vi "save_txt.vi"(8 "error in (no error)":errorcluster, 10 "Data":dbl[](array[numeric]), 11 "Path":path) -> (0 "error out":errorcluster)   [LabVIEW 2024]
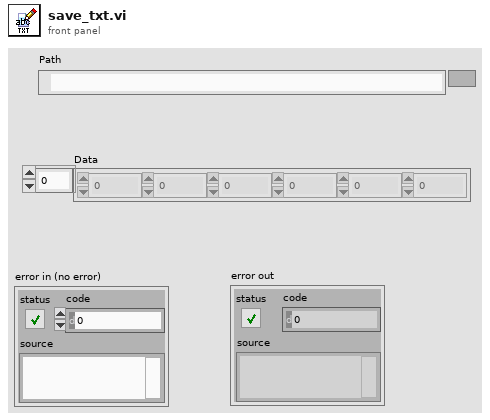
[diagram p1: front panel]
types:
  T1 = enum16{"open", "replace", "create", "open or create", "replace or create", "replace or create with confirmation"}
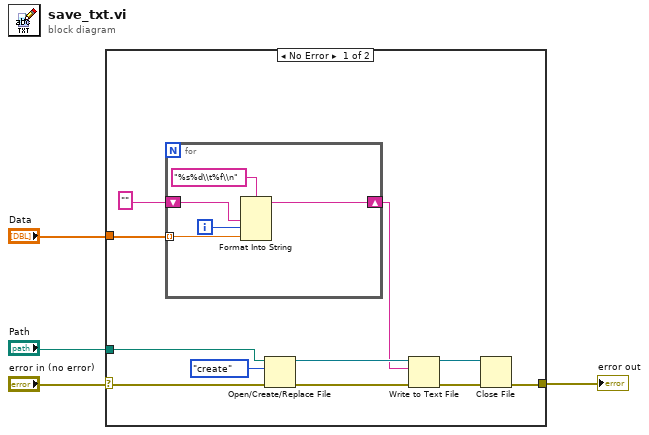
[diagram p0: block diagram]
diagram:
  n1 = case shown="No Error" "error in (no error)" {
    selector: "error in (no error)" -> [w14 w21]
    tunnel: [w11 w21] -> w3
    tunnel: "Data" -> [w15 _]
    tunnel: "Path" -> [w10 _]
    frame No Error {
      n2 = for {
        tunnel: w15 -> [w20] mode=indexing
        shift-right: [w18] -> w7
        shift-left: "" -> [w16]
        i -> [w17]
        n3 = Format Into String(format string="%s%d\\t%f\\n", w16, w17, w20) -> (resulting string=w18:string)  [unwired: 2 in, 1 out]
      }
      n4 = Open/Create/Replace File(file path (use dialog)=w10, error in=w14, operation (0:open)=T1."create") -> (refnum out=w9:refnum<file>, error out=w13:errorcluster)  [unwired: 3 in, 1 out]
      n5 = Write to Text File(file (use dialog)=w9, text=w7, error in=w13) -> (refnum out=w8:refnum<file>, error out=w12:errorcluster)  [unwired: 1 in, 1 out]
      n6 = Close File(refnum=w8, error in=w12) -> (error out=w11:errorcluster)  [unwired: 1 out]
    }
    frame Error {
    }
  }
  "error out" <- w3
